vi "CRYSetActivehalf DataView.vi"(11 "Frame nID":i32) -> ()   [LabVIEW 2013]
uses:
  CRYNew View Global.vi
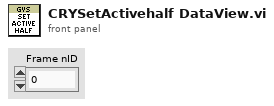
[diagram p1: front panel]
types:
  T1 = typedef "Graph Main Info Cluster.ctl" = cluster{"Selected_BarIdx":i32, "Selected_PanelIdx":i32, "Graph Main VIRef":refnum<vi>, "ToolBarClick":bool, "Spliter Ref Array":refnum<vi>[], "Panel Ref Array":refnum<vi>[], "Spliter_matrix":i32[][], "Panel_matrix":i32[][], "child_spliterIdx_matrix":i32[][], "split_pos_matrix":i32[][], "Title State":bool, "sQueueName":string, "Frame nID":i32, "Graph VIRef Array":cluster{"Graph VIRef":refnum<vi>, "Panel Idx":i32, "Frame VIRef":refnum<vi>, "Icon Ring":i32, "Graph Type":string}[], "View Type":string}
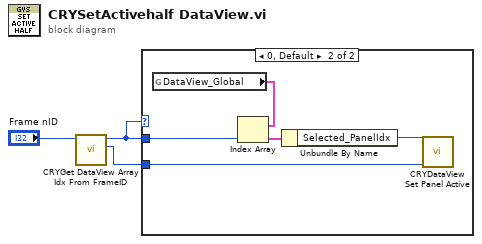
[diagram p0: block diagram]
diagram:
  n1 = call "CRYGet DataView Array Idx From FrameID.vi"("Frame nID"="Frame nID") -> ("DataView idx"=w2:i32, "DataView Array idx"=w1:i32)  [unwired: 9 in]
  n2 = case shown="0, Default" w1 {
    tunnel: w1 -> [_ w7]
    tunnel: w2 -> [_ w5]
    frame -1 {
    }
    frame 0, Default {
      n3 = global read "CRYNew View Global.vi" "DataView_Global"() -> (w8:T1[])
      n4 = Index Array(array=w8, index=w7) -> (element=w6:T1)
      n5 = Unbundle By Name(w6) -> ("Selected_PanelIdx"=w4:i32)
      n6 = call "CRYDataView Set Panel Active.vi"("DataView Index"=w5, "Selected Panel Idx In"=w4) -> ()  [unwired: 10 in]
    }
  }
